vi "ToTable Test.vi"() -> (0 "error out":errorcluster)   [LabVIEW 2015, in "Increment tests.lvlib"]
doc: "Tests the 'To Table' method."
uses:
  Increment tests.lvlib
  <vilib>/NI/Module Execution Interface/Engine Configuration/engine configuration.lvclass
  editor node/Increment editor node.lvclass
  <vilib>/NI/Tag Bus/tag/tag descriptor.lvclass
  <vilib>/NI/Tag Bus/tag/tag descriptor.lvclass/tag descriptor.ctl
  <vilib>/NI/Configuration Framework/serializable configuration/NISE_CEF_serializable configuration.lvclass/NISE_CEF_serializable configuration.ctl
  <vilib>/Utility/LVClass/Get LV Class Name.vi
  <vilib>/NI/Configuration Framework/error generator/NISE_error generator.vi
  <vilib>/NI/Configuration Framework/serializable configuration/NISE_CEF_serializable configuration.lvclass
panel:
  out "table":string[][](array[string])
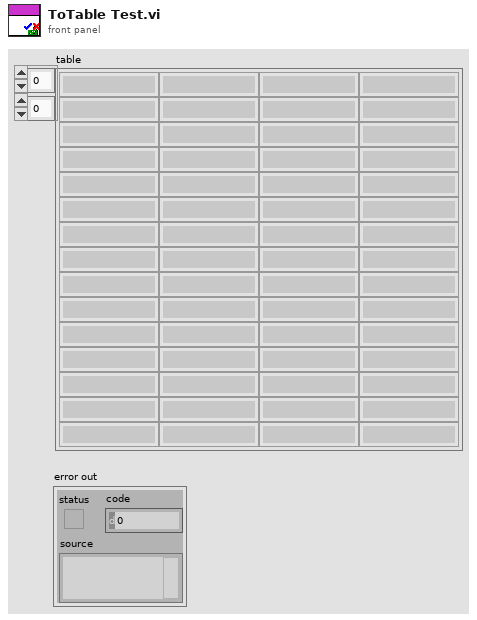
[diagram p1: front panel]
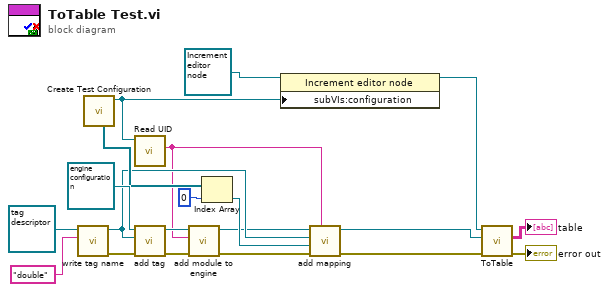
[diagram p0: block diagram]
diagram:
  n1 = call <vilib>:"write tag name.vi"("name"="double", "system tag in"=refnum<class "tag descriptor.lvclass"> refnum ("tag descriptor")) -> ("error out"=w1:errorcluster, "system tag out"=w10:refnum<class "tag descriptor.lvclass">)  [unwired: 8 in]
  n2 = call "Create Test Configuration.vi"() -> ("Module Configuration"=w9:refnum<class "Increment configuration.lvclass">, "Channels"=w13:refnum<class "TBM channel.lvclass">[])  [unwired: 6 in, 4 out]
  n3 = call <vilib>:"Read UID.vi"("configuration in"=w9) -> ("instance id"=w5:string)  [unwired: 8 in, 2 out]
  n4 = call-dynamic "add tag.vi"("error in"=w1, "tag descriptor"=w10, "engine configuration in"=refnum<class "engine configuration.lvclass"> refnum ("engine configuration")) -> ("error out"=w2:errorcluster, "engine configuration out"=w7:refnum<class "engine configuration.lvclass">)  [unwired: 7 in]
  n5 = call-dynamic "add module to engine.vi"("error in"=w2, "module ID"=w5, "engine configuration in"=w7) -> ("error out"=w4:errorcluster, "engine configuration out"=w6:refnum<class "engine configuration.lvclass">)  [unwired: 7 in]
  n6 = Index Array(array=w13, index=0) -> (element=w11:refnum<class "TBM channel.lvclass">)
  n7 = property class="Increment editor node"(reference=refnum<class "Increment editor node.lvclass"> refnum ("node in"), "subVIs:configuration"=w9) -> (reference out=w19:refnum<class "Increment editor node.lvclass">)  [unwired: 1 in, 1 out]
  n8 = call-dynamic "add mapping.vi"("owner ID"=w5, "error in"=w4, "channel"=w11, "tag descriptor"=w10, "engine configuration"=w6) -> ("error out"=w3:errorcluster, "engine configuration out"=w8:refnum<class "engine configuration.lvclass">)  [unwired: 5 in]
  n9 = call-dynamic "ToTable.vi"("error in"=w3, "variant"=w8, "Increment editor node in"=w19) -> ("error out"=→"error out":errorcluster, "table"=→"table":string[][])  [unwired: 5 in, 2 out]
